vi "Interpoints.vi"(10 "Min_dist":dbl, 11 "reference_corners":dbl[][](array[numeric])) -> (2 "Corners":dbl[][](array[numeric]), 3 "Reference path":dbl[][](array[numeric]))   [LabVIEW 2015]
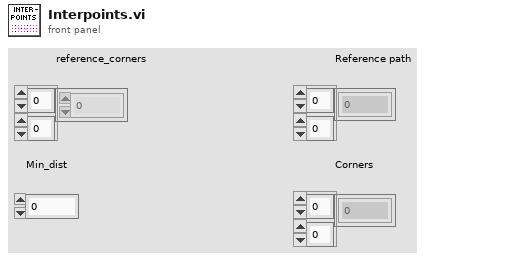
[diagram p1: front panel]
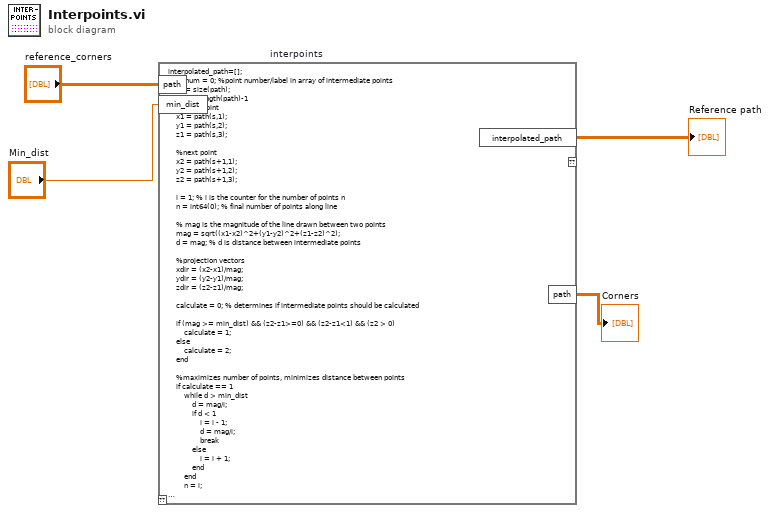
[diagram p0: block diagram]
diagram:
  n1 = script code="interpolated_path=[];\npointnum = 0; %point number/label in array of intermediate points\n[r,c] = size(path);\nfor s = 1:length(path)-1\n    %start point\n    x1 = path(s,1);\n    y1 = path(s,2);\n    z1 = path(s,3);\n    \n    %next point\n    x2 = path(s+1,1);\n    y2 = path(s+1,2); \n    z2 = path(s+1,3);\n\n    i = 1; % i is the counter for the number of points n\n    n = int64(0); % final number of points along line\n    \n    % mag is the magnitude of the line drawn between two points\n    mag = sqrt((x1-x2)^2+(y1-y2)^2+(z1-z2)^2);\n    d = mag; % d is distance between intermediate points\n    \n    %projection vectors\n    xdir = (x2-x1)/mag;\n    ydir = (y2-y1)/mag;\n    zdir = (z2-z1)/mag;\n\n    calculate = 0; % determines if intermediate points should be calculated\n\n    if (mag >= min_dist) && (z2-z1>=0) && (z2-z1<1) && (z2 > 0)\n        calculate = 1;\n    else\n        calculate = 2;\n    end\n    \n    %maximizes number of points, minimizes distance between points\n    if calculate == 1\n        while d > min_dist\n            d = mag/i;\n            if d < 1\n                i = i - 1;\n                d = mag/i;\n                break\n            else\n                i = i + 1;\n            end\n        end\n        n = i;\n\n        %point number, x coord, y coord, z coord\n        count = 0;\n        while count < n-1\n            pointnum = pointnum + 1;\n            count = count + 1;\n            interpolated_path(pointnum, 1) = x1+(xdir*(count-1)*d);\n            interpolated_path(pointnum, 2) = y1+(ydir*(count-1)*d);\n            interpolated_path(pointnum, 3) = z1+(zdir*(count-1)*d);\n        end\n\n    elseif calculate == 2\n        pointnum = pointnum + 1;\n        interpolated_path(pointnum, 1) = x1;\n        interpolated_path(pointnum, 2) = y1;\n        interpolated_path(pointnum, 3) = z1;\n    end\nend\n% store last point in path to path MATRIX\ninterpolated_path(end+1, 1) = path(r,1);\ninterpolated_path(end, 2) = path(r,2);\ninterpolated_path(end, 3) = path(r,3);" "interpoints"("min_dist"="Min_dist", "path"="reference_corners") -> ("interpolated_path"=→"Reference path":dbl[][], "path"=→"Corners":dbl[][])  [unwired: 1 in, 1 out]
